vi "ERD_Write_SLB.vi"(0 "GEA2 Reference In":refnum<k24>, 5 "GEA Inputs":T3={"Source"=228, "Destination"=36} {"Destination" format="%.0x"; "Source" format="%.0x"}, 7 "Write ERD List":T1[](array[typedef]) {"ERD Number" format="%.0x"}, 11 "Error In":errorcluster) -> (4 "GEA2 Reference Out":refnum<k24>, 15 "Error Out":errorcluster)   [LabVIEW 2016]
uses:
  Common/LabVIEW GEA2 Toolkit/LabVIEW_GEA2_Toolkit.lvlibp/type defs/Source_Destination.ctl
  Common/LabVIEW GEA2 Toolkit/LabVIEW_GEA2_Toolkit.lvlibp/type defs/ERD Write Data In.ctl
  Common/LabVIEW GEA2 Toolkit/LabVIEW_GEA2_Toolkit.lvlibp/type defs/Data Type.ctl
  Q:/Common/DLLs/GEA3/GeaCommunication.dll
  Common/DLLs/GEA3/GeaCommunication.dll
  Common/LabVIEW GEA2 Toolkit/LabVIEW_GEA2_Toolkit.lvlibp
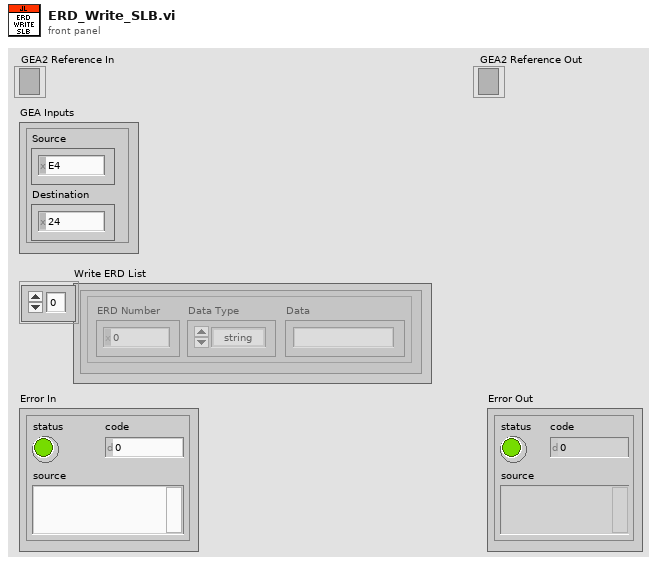
[diagram p1: front panel]
types:
  T1 = typedef "LabVIEW_GEA2_Toolkit.lvlibp/ERD Write Data In.ctl" = cluster{"ERD Number":u16, "Data Type":T2, "Data":string}
  T2 = typedef "LabVIEW_GEA2_Toolkit.lvlibp/Data Type.ctl" = enum16{"string", "boolean", "uint8_t", "uint16_t", "uint32_t", "uint64_t", "int8_t", "int16_t", "int32_t", "int64_t"}
  T3 = typedef "LabVIEW_GEA2_Toolkit.lvlibp/Source_Destination.ctl" = cluster{"Source":u8, "Destination":u8}
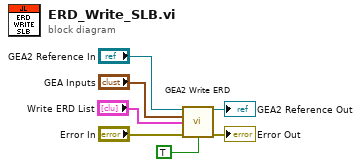
[diagram p0: block diagram]
diagram:
  n1 = call "GEA2 Write ERD.vi"("GEA2 Reference In"="GEA2 Reference In", "GEA Inputs"="GEA Inputs", "Write ERD List"="Write ERD List", "Error In"="Error In", "Verify ERD Response?"=TRUE) -> ("GEA2 Reference Out"=→"GEA2 Reference Out":refnum<k24>, "Error Out"=→"Error Out":errorcluster)  [unwired: 8 in, 1 out]
